vi "SQL_Table_Test_SelectByTime.vi"() -> ()   [LabVIEW 2014]
panel:
  in  "时间标识":timestamp
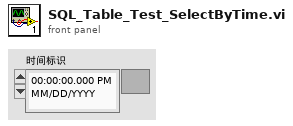
[diagram p1: front panel]
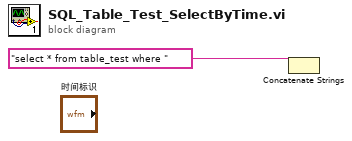
[diagram p0: block diagram]
diagram:
  n1 = Concatenate Strings("select * from table_test where " ("Command Text")) -> ()  [unwired: 1 in, 1 out]
